vi "afmmode.vi"() -> ()   [LabVIEW 2017]
uses:
  Program Files/National Instruments/LabVIEW 2019/user.lib/HapticSTM/HapticSTM.lvlib
  Program Files/National Instruments/LabVIEW 2019/user.lib/Nanonis Prog Interface V5/Nanonis Prog Interface.lvlib
panel:
  out "force":dbl
  out "Z Write (m) 2":dbl
  in  "Z Write?":bool
  in  "Save":bool
  in  "# Sample Points":i32=4096
  out "Signal value":sgl format="%#_6p"
  out "Z Write (m)":dbl
  in  "Signal index (0-127)":i8
  in  "Upper Limit (mm)":dbl=50.0
  in  "Lower Limit (mm)":dbl=-40.0
  in  "Upper Limit (nm)":dbl=1.0
  in  "Lower Limit (nm)":dbl
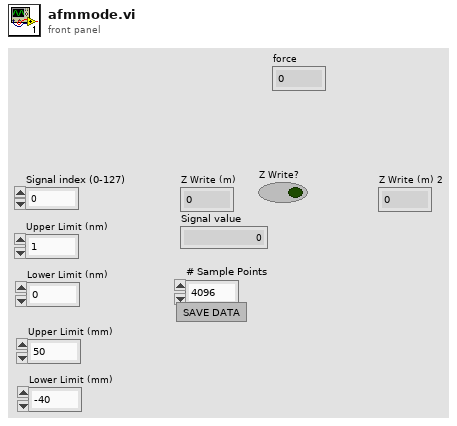
[diagram p1: front panel]
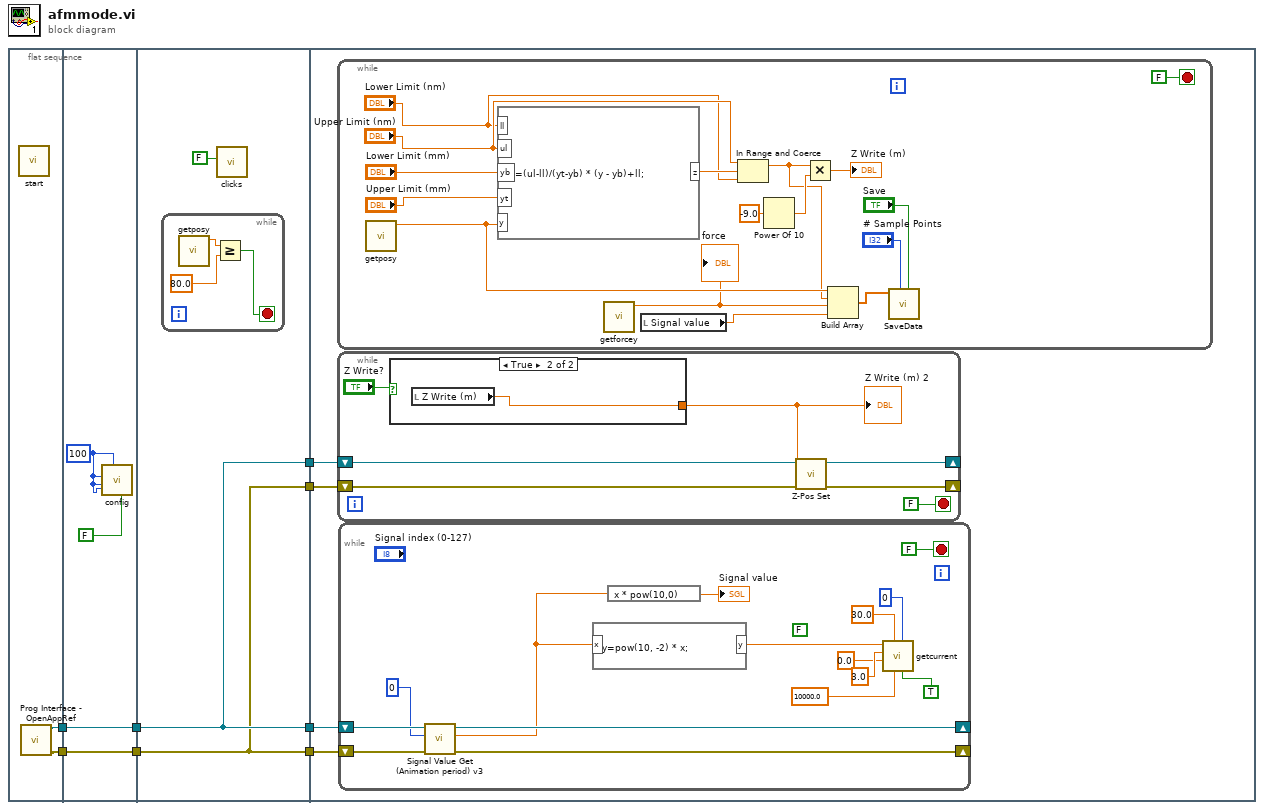
[diagram p0: block diagram]
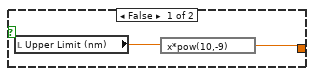
[diagram p2: hidden frame]
diagram:
  n1 = flat-sequence {
    tunnel: [w10] -> w8
    tunnel: [w9] -> w3
    tunnel: w8 -> [w12]
    tunnel: [w12] -> w7
    tunnel: [w11] -> w4
    tunnel: w3 -> [w11]
    tunnel: w7 -> [w16]
    tunnel: [w16] -> w6
    tunnel: [w15] -> w5
    tunnel: w4 -> [w15]
    tunnel: [w16] -> w2
    tunnel: [w15] -> w1
    tunnel: w6 -> [w24]
    tunnel: w5 -> [w23]
    tunnel: w2 -> [w22]
    tunnel: w1 -> [w21]
    frame #0 {
      n2 = call "start.vi"() -> ()  [unwired: 11 in, 1 out]
      n3 = call <userlib>:"Prog Interface - OpenAppRef.vi"() -> ("Error out"=w9:errorcluster, "Application reference"=w10:refnum<vi>)  [unwired: 6 in]
    }
    frame #1 {
      w13 = 100 ("sizeofimgx")
      n4 = call "config.vi"("feedback"=FALSE, "sizeofimgz"=w13, "sizeofimgx"=w13, "scopez"=w13, "scopex"=w13) -> ()  [unwired: 7 in]
    }
    frame #2 {
      n5 = while {
        stop <- w18 stop-if-true
        n6 = call "getposy.vi"() -> ("function return"=w20:dbl)  [unwired: 11 in]
        n7 = Greater Or Equal?(x=w20, y=80.0) -> (x >= y?=w18:bool)
      }
      n8 = call "clicks.vi"("planing"=FALSE) -> ()  [unwired: 10 in, 1 out]
    }
    frame #3 {
      n9 = while {
        stop <- FALSE stop-if-true
        n10 = call "getposy.vi"() -> ("function return"=w56:dbl)  [unwired: 11 in]
        n11 = formula code="z =(ul-ll)/(yt-yb) * (y - yb)+ll;"("ll"="Lower Limit (nm)", "ul"="Upper Limit (nm)", "yb"="Lower Limit (mm)", "yt"="Upper Limit (mm)", "y"=w56) -> ("z"=w60:dbl)
        n12 = call "getforcey.vi"() -> ("function return"=w54:dbl)  [unwired: 11 in]
        "force" <- w54
        n13 = local read "Signal value"() -> (w51:sgl)
        n14 = In Range and Coerce(upper limit="Upper Limit (nm)", x=w60, lower limit="Lower Limit (nm)") -> (coerced(x)=w55:dbl)  [unwired: 1 out]
        n15 = Power Of 10(x=-9.0) -> (10^x=w61:dbl)
        n16 = Multiply(x=w55, y=w61) -> (x*y=→"Z Write (m)":dbl)
        n17 = Build Array(w56, w55, w54, w51) -> (w50:dbl[])
        n18 = call "SaveData.vi"("Save"="Save", "# Sample Points"="# Sample Points", "Data"=w50) -> ()  [unwired: 9 in]
      }
      n19 = while {
        shift-right: [w27] -> _
        shift-left: w22 -> [w29]
        shift-right: [w26] -> _
        shift-left: w21 -> [w28]
        stop <- FALSE stop-if-true
        n20 = case shown="True" "Z Write?" {
          tunnel: [w32 w34] -> w25
          frame False {
            n21 = local read "Upper Limit (nm)"() -> (w33:dbl)
            n22 = expression code="x*pow(10,-9)"(w33) -> (w32:dbl)
          }
          frame True {
            n23 = local read "Z Write (m)"() -> (w34:dbl)
          }
        }
        "Z Write (m) 2" <- w25
        n24 = call <userlib>:"Z-Pos Set.vi"("error in (no error)"=w28, "Z position (m)"=w25, "Application ref in"=w29) -> ("error out"=w26:errorcluster, "Application ref out"=w27:refnum<vi>)  [unwired: 7 in]
      }
      n25 = while {
        shift-right: [w39] -> _
        shift-left: w24 -> [w41]
        shift-right: [w38] -> _
        shift-left: w23 -> [w40]
        stop <- FALSE stop-if-true
        (unwired) FALSE ("feedback")
        n26 = call <userlib>:"Signal Value Get (Animation period) v3.vi"("error in (no error)"=w40, "Signal index (0-127)"=i8 0, "Application ref in"=w41) -> ("error out"=w38:errorcluster, "Signal value"=w35:sgl, "Application ref out"=w39:refnum<vi>)  [unwired: 5 in]
        n27 = formula code="y=pow(10, -2) * x;"("x"=w35) -> ("y"=w42:dbl)
        n28 = expression code="x * pow(10,0)"(w35) -> (→"Signal value":sgl)
        n29 = call "getcurrent.vi"("afmmode"=TRUE, "forcemode"=0, "maxcurrentin"=10000.0, "setpoint"=30.0, "minforcey"=0.0, "maxforcey"=3.0, "currentin"=w42) -> ()  [unwired: 5 in]
      }
    }
  }
